vi "Add Default Menu.vi"(8 "error in":errorcluster, 11 "Path":path) -> (0 "error out":errorcluster)   [LabVIEW 2010]
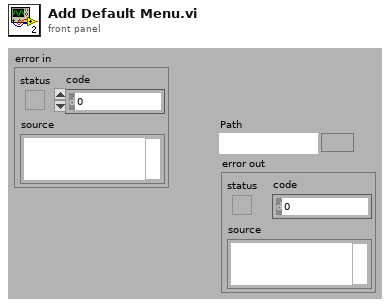
[diagram p1: front panel]
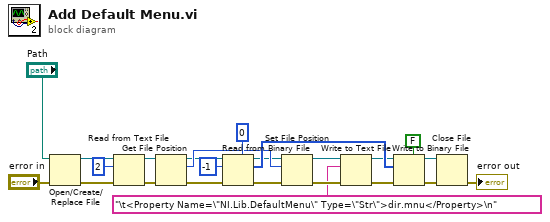
[diagram p0: block diagram]
diagram:
  n1 = Open/Create/Replace File(file path (use dialog)="Path", error in="error in") -> (refnum out=w4:refnum<file>, error out=w5:errorcluster)  [unwired: 4 in, 1 out]
  n2 = Read from Text File(file (use dialog)=w4, count=2, error in=w5) -> (refnum out=w13:refnum<file>, error out=w12:errorcluster)  [unwired: 1 in, 2 out]
  n3 = Get File Position(4:w12, 7:w13) -> (0:w15:errorcluster, 2:w20:i64, 3:w14:refnum<file>)
  n4 = Read from Binary File(5:u8 0, 8:w15, 10:-1 ("count (1)"), 11:w14) -> (0:w17:errorcluster, 2:w23:u8[], 3:w16:refnum<file>)  [unwired: 2 in, 1 out]
  n5 = Set File Position(offset (in bytes) (0)=w20, refnum=w16, error in=w17) -> (refnum out=w19:refnum<file>, error out=w18:errorcluster)  [unwired: 1 in]
  n6 = Write to Text File(file (use dialog)=w19, text="\t<Property Name=\"NI.Lib.DefaultMenu\" Type=\"Str\">dir.mnu</Property>\n", error in=w18) -> (refnum out=w8:refnum<file>, error out=w9:errorcluster)  [unwired: 1 in, 1 out]
  n7 = Write to Binary File(file (use dialog)=w8, data=w23, error in=w9, 5:FALSE ("prepend array or string size? (T)")) -> (refnum out=w10:refnum<file>, error out=w11:errorcluster)  [unwired: 2 in, 1 out]
  n8 = Close File(refnum=w10, error in=w11) -> (error out=→"error out":errorcluster)  [unwired: 1 out]
